vi "Rozbicie tekstu na współrzędną w formacie  DMS.vi"(7 "Współrzędna tekstowa":string) -> (0 "Kierunek":string, 1 "Druga współrzędna":string, 2 "S":dbl, 3 "M":dbl, 5 "D":dbl)   [LabVIEW 2012, in "Biblioteka moduł map v3.lvlib" / "Konwersja wsp.lvlib" / "Wyciągnięcie z tekstu współrzędnej.lvlib"]
doc: "SubVI ma za zadanie odfiltorać ze współrzędnej tekstowej takie wartości jak stopnie, minuty, sekundy oraz kierunek. Na wyjściu podaje również drugą współrzędną w postaci tekstowej, którą należy później odfiltrować."
uses:
  <vilib>/regexp/Match Regular Expression.xnode
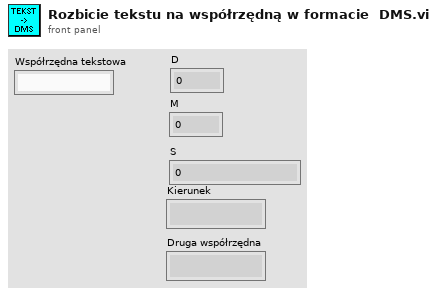
[diagram p1: front panel]
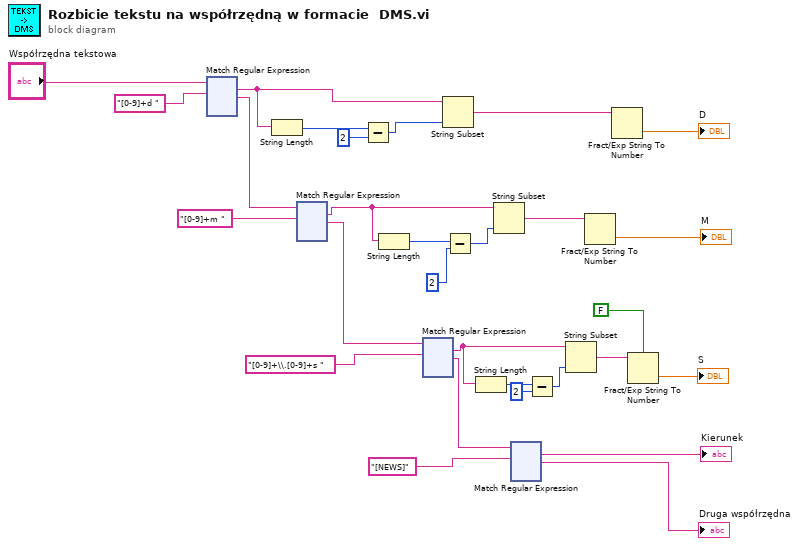
[diagram p0: block diagram]
diagram:
  n1 = xnode "Match Regular Expression"("input string"="Współrzędna tekstowa", "regular expression"="[0-9]+d ") -> ("whole match"=w11:string, "after match"=w13:string)  [unwired: 4 in, 3 out]
  n2 = String Length(string=w11) -> (length=w21:i32)
  n3 = xnode "Match Regular Expression"("input string"=w13, "regular expression"="[0-9]+m ") -> ("whole match"=w14:string, "after match"=w15:string)  [unwired: 4 in, 3 out]
  n4 = Subtract(x=w21, y=2) -> (x-y=w23:i32)
  n5 = String Length(string=w14) -> (length=w26:i32)
  n6 = xnode "Match Regular Expression"("input string"=w15, "regular expression"="[0-9]+\\.[0-9]+s ") -> ("whole match"=w17:string, "after match"=w18:string)  [unwired: 4 in, 3 out]
  n7 = String Subset(string=w11, length (rest)=w23) -> (substring=w6:string)  [unwired: 1 in]
  n8 = Subtract(x=w26, y=2) -> (x-y=w24:i32)
  n9 = String Length(string=w17) -> (length=w27:i32)
  n10 = String Subset(string=w14, length (rest)=w24) -> (substring=w4:string)  [unwired: 1 in]
  n11 = xnode "Match Regular Expression"("input string"=w18, "regular expression"="[NEWS]") -> ("whole match"=→"Kierunek":string, "after match"=→"Druga współrzędna":string)  [unwired: 4 in, 3 out]
  n12 = Subtract(x=w27, y=2) -> (x-y=w28:i32)
  n13 = String Subset(string=w17, length (rest)=w28) -> (substring=w9:string)  [unwired: 1 in]
  n14 = Fract/Exp String To Number(string=w4) -> (number=→"M":dbl)  [unwired: 3 in, 1 out]
  n15 = Fract/Exp String To Number(string=w6) -> (number=→"D":dbl)  [unwired: 3 in, 1 out]
  n16 = Fract/Exp String To Number(use system decimal point (T)=FALSE, string=w9) -> (number=→"S":dbl)  [unwired: 2 in, 1 out]
